vi "Create RT FIFOs.vi"(6 "FIFO Idx Qs":T5, 8 "error in (no error)":errorcluster, 11 "Label Transfer Config":T1 {"Block Data Refs"."Data Reference" format="%.0x"}) -> (0 "error out":errorcluster, 3 "output cluster":T4)   [LabVIEW 2012, in "AIT 429 Engine.lvlib"]
uses:
  AIT 429 Engine.lvlib
  RT Controls/FIFO Idx Qs.ctl
  RT Controls/FIFO.ctl
  RT Controls/Label Transfer Config.ctl
  <vilib>/NI Veristand/Custom Device API/Block Data Reference.ctl
  <vilib>/NI Veristand/Custom Device API/Data Reference.ctl
  RT Controls/Data Ref FGV Command.ctl
  <vilib>/NI Veristand/Custom Device API/Custom Device API.lvlib
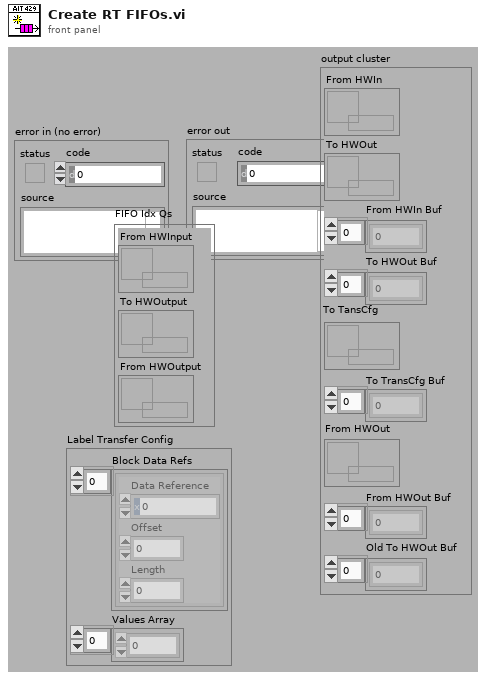
[diagram p1: front panel]
types:
  T1 = typedef "AIT 429 Engine.lvlib/Label Transfer Config.ctl" = cluster{"Block Data Refs":T2[], "Values Array":dbl[]}
  T2 = typedef "Custom Device API.lvlib/Block Data Reference.ctl" = cluster{"Data Reference":T3, "Offset":i32, "Length":i32}
  T3 = typedef "Custom Device API.lvlib/Data Reference.ctl" = i32
  T4 = typedef "AIT 429 Engine.lvlib/FIFO.ctl" = cluster{"From HWIn":refnum<k33>, "To HWOut":refnum<k33>, "From HWIn Buf":dbl[], "To HWOut Buf":dbl[], "To TansCfg":refnum<k33>, "To TransCfg Buf":dbl[], "From HWOut":refnum<k33>, "From HWOut Buf":dbl[], "Old To HWOut Buf":dbl[]}
  T5 = typedef "AIT 429 Engine.lvlib/FIFO Idx Qs.ctl" = cluster{"From HWInput":refnum<queue>, "To HWOutput":refnum<queue>, "From HWOutput":refnum<queue>}
  T6 = typedef "AIT 429 Engine.lvlib/Data Ref FGV Command.ctl" = enum16{"Intialize", "Get", "Update"}
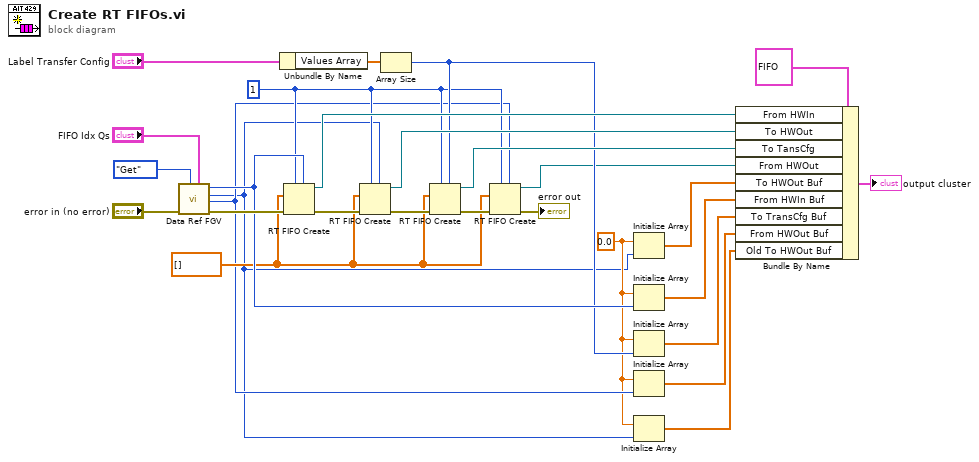
[diagram p0: block diagram]
diagram:
  w3 = 0.0
  w8 = dbl[] []
  w7 = u32 1 ("size (10)")
  n1 = call "Data Ref FGV.vi"("FIFO Idx Qs"="FIFO Idx Qs", "Command"=Data_Ref_FGV_Command."Get", "error in (no error)"="error in (no error)") -> ("error out"=w27:errorcluster, "From HWOutput FIFO Index / Length"=w5:i32, "To HWOutput FIFO Index / Length"=w2:i32, "From HWInput FIFO Index / Length"=w24:i32)  [unwired: 5 in]
  n2 = Unbundle By Name("Label Transfer Config") -> ("Values Array"=w15:dbl[])
  n3 = RT FIFO Create(1:w8, 3:w27, 4:w7, 6:w24) -> (8:w21:refnum<k33>, 11:w25:errorcluster)  [unwired: 4 in, 1 out]
  n4 = RT FIFO Create(1:w8, 3:w25, 4:w7, 6:w2) -> (8:w20:refnum<k33>, 11:w14:errorcluster)  [unwired: 4 in, 1 out]
  n5 = Array Size(array=w15) -> (size(s)=w12:i32)
  n6 = RT FIFO Create(1:w8, 3:w14, 4:w7, 6:w12) -> (8:w13:refnum<k33>, 11:w9:errorcluster)  [unwired: 4 in, 1 out]
  n7 = RT FIFO Create(1:w8, 3:w9, 4:w7, 6:w5) -> (8:w4:refnum<k33>, 11:→"error out":errorcluster)  [unwired: 4 in, 1 out]
  n8 = Initialize Array(w3, w2) -> (w19:dbl[])
  n9 = Initialize Array(w3, w24) -> (w18:dbl[])
  n10 = Initialize Array(w3, w12) -> (w11:dbl[])
  n11 = Initialize Array(w3, w5) -> (w10:dbl[])
  n12 = Initialize Array(w3, w2) -> (w1:dbl[])
  n13 = Bundle By Name(cluster=T4 {"From HWIn"=refnum, "To HWOut"=refnum, "From HWIn Buf"=[], "To HWOut Buf"=[], "To TansCfg"=refnum, "To TransCfg Buf"=[], "From HWOut"=refnum, "From HWOut Buf"=[], "Old To HWOut Buf"=[]} ("FIFOs"), "From HWIn"=w21, "To HWOut"=w20, "To TansCfg"=w13, "From HWOut"=w4, "To HWOut Buf"=w19, "From HWIn Buf"=w18, "To TransCfg Buf"=w11, "From HWOut Buf"=w10, "Old To HWOut Buf"=w1) -> (→"output cluster":T4)
